vi "Read write Master.vi"(8 "error in (no error)":errorcluster, 10 "ELAN data unit in":refnum<class "SMSD Data Unit.lvclass">, 11 "ELAN master in":refnum<class "SMSD Master.lvclass">) -> (0 "error out":errorcluster, 1 "PDU valid?":bool, 2 "ELAN data unit out":refnum<class "SMSD Data Unit.lvclass">, 3 "ELAN master out":refnum<class "SMSD Master.lvclass">)   [LabVIEW 2021, in "SMSD Master.lvclass"]
doc: "This VI allows a mutex for the master API without restricting any other functions. This mutex is currently unimplemented."
uses:
  SMSD Master.lvclass
  Data Unit/SMSD Data Unit/SMSD Data Unit.lvclass
  SMSD Master.lvclass/SMSD Master.ctl
  Transmission Data Unit/SMSD/SMSD ADU.lvclass/SMSD ADU.ctl
  Data Unit/SMSD Data Unit/SMSD Data Unit.lvclass/SMSD Data Unit.ctl
  Modbus_v121c/Network Interface/TCP Interface/TCP Shared Components/TCP Write.vi
  Data Unit/SMSD Data Unit/Flatten PDU.vi
  Data Unit/SMSD Data Unit/Unflatten to PDU.vi
  Modbus_v121c/Network Interface/TCP Interface/TCP Shared Components/TCP Read.vi
  <vilib>/Utility/error.llb/Clear Errors.vi
  Transmission Data Unit/SMSD/SMSD ADU.lvclass
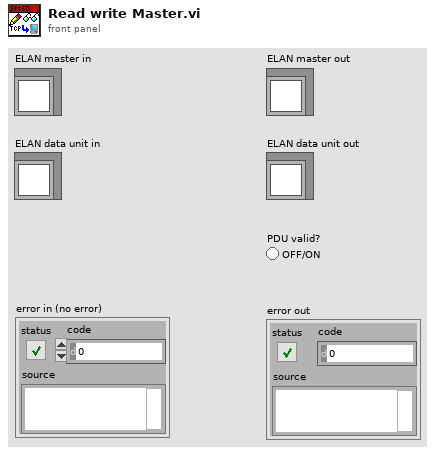
[diagram p1: front panel]
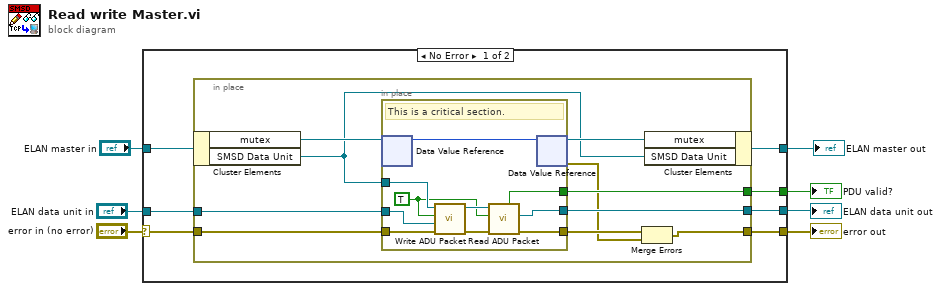
[diagram p0: block diagram]
diagram:
  n1 = case shown="No Error" "error in (no error)" {
    selector: "error in (no error)" -> [w9 w35]
    tunnel: "ELAN master in" -> [w10 w36]
    tunnel: [w8 w36] -> w6
    tunnel: "ELAN data unit in" -> [w14 w37]
    tunnel: [w13 w37] -> w4
    tunnel: [w12 w35] -> w3
    tunnel: [w11 _] -> w2
    frame No Error {
      n2 = in-place {
        in-place-border: w9 -> [w23]
        in-place-border: w14 -> [w22]
        in-place-border: [w20] -> w13
        in-place-border: [w19] -> w12
        in-place-border: [w18] -> w11
        n3 = in-place-cluster #1(w10) -> ("mutex"=w24:refnum<data-value>, "SMSD Data Unit"=w15:refnum<class "SMSD ADU.lvclass">)
        n4 = in-place {
          in-place-border: w23 -> [w31]
          in-place-border: w22 -> [w30]
          in-place-border: [w26] -> w17
          in-place-border: [w25] -> w20
          in-place-border: [w29] -> w18
          in-place-border: w15 -> [w28]
          w27 = TRUE ("isMaster (f)")
          # "This is a critical section."
          n5 = in-place-dvr #2(w24) -> (w32:u8)  [unwired: 1 out]
          n6 = call "Write ADU Packet.vi"("error in"=w31, "SMSD Data Unit"=w30, "isMaster (f)"=w27, "IP simple ADU in"=w28) -> ("error out"=w34:errorcluster, "IP simple ADU out"=w33:refnum<class "SMSD ADU.lvclass">)  [unwired: 6 in]
          n7 = call "Read ADU Packet.vi"("error in"=w34, "isMaster (f)"=w27, "IP simple ADU in"=w33) -> ("error out"=w26:errorcluster, "SMSD data unit out"=w25:refnum<class "SMSD Data Unit.lvclass">, "PDU Valid?"=w29:bool)  [unwired: 5 in, 1 out]
          n8 = in-place-dvr #2(w32) -> (w21:refnum<data-value>, w16:errorcluster)
        }
        n9 = Merge Errors(w17, w16) -> (w19:errorcluster)
        n10 = in-place-cluster #1("mutex"=w21, "SMSD Data Unit"=w15) -> (w8:refnum<class "SMSD Master.lvclass">)
      }
    }
    frame Error {
    }
  }
  "ELAN data unit out" <- w4
  "ELAN master out" <- w6
  "error out" <- w3
  "PDU valid?" <- w2
